vi "ButtonRecieve.vi"(8 "error in (no error)":errorcluster, 11 "Notifier Name":string="Joystick") -> (0 "error out":errorcluster, 2 "notification":i8)   [LabVIEW 2013]
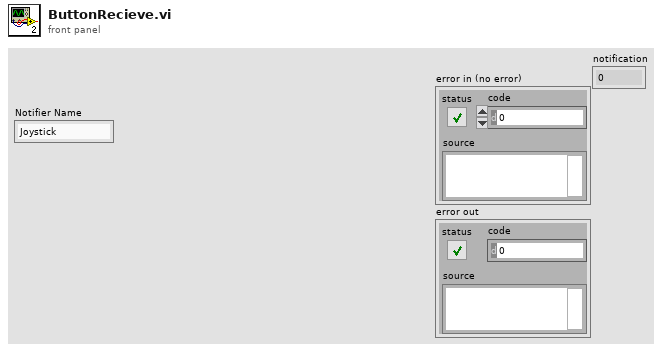
[diagram p1: front panel]
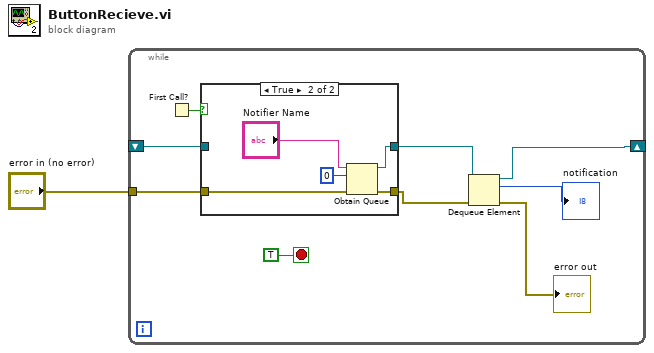
[diagram p0: block diagram]
diagram:
  n1 = while {
    shift-right: [w2] -> _
    shift-left: _ -> [w7]
    tunnel: "error in (no error)" -> [w8]
    stop <- TRUE stop-if-true
    n2 = First Call?() -> (First Call?: T/F=w9:bool)
    n3 = case shown="True" w9 {
      tunnel: [w12 w14] -> w6
      tunnel: w8 -> [w11 w15]
      tunnel: w7 -> [w12 _]
      tunnel: [w11 w13] -> w5
      frame False {
      }
      frame True {
        n4 = Obtain Queue(name (unnamed)="Notifier Name", element data type=i8 0, error in (no error)=w15) -> (queue out=w14:refnum<queue>, error out=w13:errorcluster)  [unwired: 2 in, 1 out]
      }
    }
    n5 = Dequeue Element(queue=w6, error in (no error)=w5) -> (queue out=w2:refnum<queue>, element=→"notification":i8, error out=→"error out":errorcluster)  [unwired: 1 in, 1 out]
  }
